vi "Remove Test.vi"(7 "Test ID":string, 8 "error in (no error)":errorcluster, 11 "Test Executive Ref":refnum<data-value>) -> (0 "error out":errorcluster, 2 "Orphaned Pointer IDs":string[](array[string]), 3 "Test Executive Ref out":refnum<data-value>)   [LabVIEW 2019, in "Test Executive.lvlib" / "TestExecutive Ref.lvclass"]
uses:
  <vilib>/gpm_packages/@cs/test-executive/Source/Test Executive/TestExecutive Ref/TestExecutive Ref.lvclass
  <vilib>/gpm_packages/@cs/test-executive/Source/Test Executive/ITestExecutive/ITest Executive.lvclass
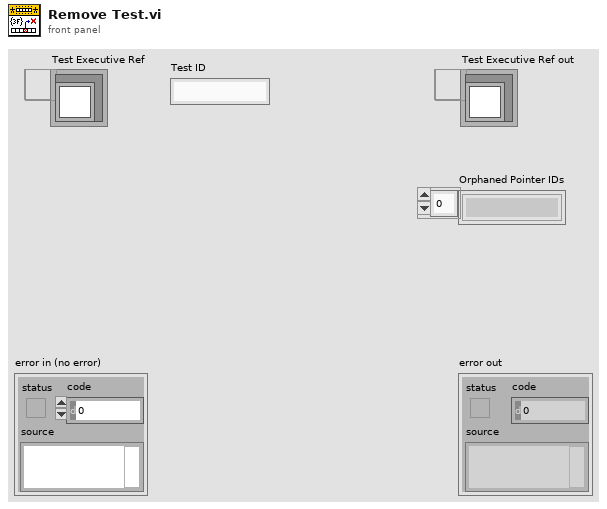
[diagram p1: front panel]
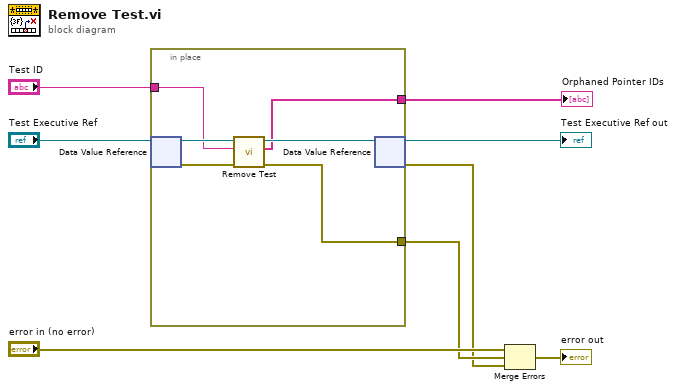
[diagram p0: block diagram]
diagram:
  n1 = in-place {
    in-place-border: "Test ID" -> [w10]
    in-place-border: [w11] -> w4
    in-place-border: [w9] -> w1
    n2 = in-place-dvr #1("Test Executive Ref") -> (w14:refnum<class "ITest Executive.lvclass">, w12:errorcluster)
    n3 = call-dynamic "Remove Test.vi"("error in (no error)"=w12, "Unique ID"=w10, "ITest Executive in"=w14) -> ("error out"=w11:errorcluster, "Orphaned Pointer IDs"=w9:string[], "ITest Executive out"=w13:refnum<class "ITest Executive.lvclass">)  [unwired: 6 in]
    n4 = in-place-dvr #1(w13) -> (→"Test Executive Ref out":refnum<data-value>, w3:errorcluster)
  }
  "Orphaned Pointer IDs" <- w1
  n5 = Merge Errors("error in (no error)", w4, w3) -> (→"error out":errorcluster)
